vi "Main.vi"   [LabVIEW 2017]
types:
  T1 = cluster{"Note Freq":dbl[], "Note Length":dbl[], "Rest":dbl[]}
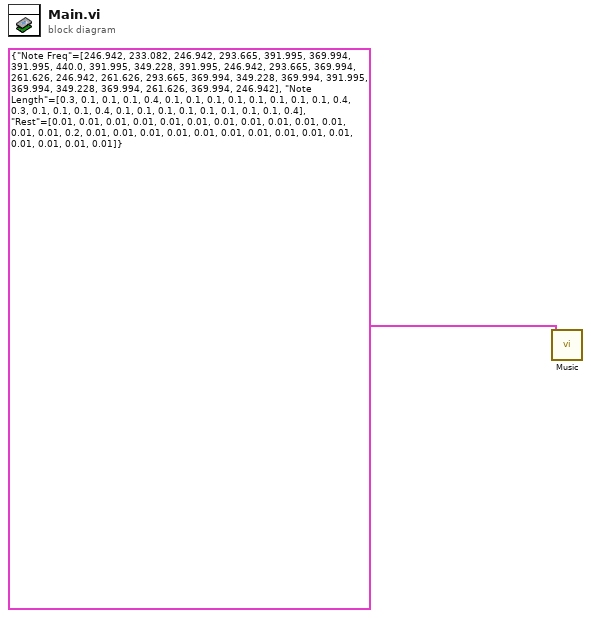
[diagram p0: block diagram]
diagram:
  n1 = call "Music.vi"(11:T1 {"Note Freq"=[246.942, 233.082, 246.942, 293.665, 391.995, 369.994, 391.995, 440.0, 391.995, 349.228, 391.995, 246.942, 293.665, 369.994, 261.626, 246.942, 261.626, 293.665, 369.994, 349.228, 369.994, 391.995, 369.994, 349.228, 369.994, 261.626, 369.994, 246.942], "Note Length"=[0.3, 0.1, 0.1, 0.1, 0.4, 0.1, 0.1, 0.1, 0.1, 0.1, 0.1, 0.1, 0.1, 0.4, 0.3, 0.1, 0.1, 0.1, 0.4, 0.1, 0.1, 0.1, 0.1, 0.1, 0.1, 0.1, 0.1, 0.4], "Rest"=[0.01, 0.01, 0.01, 0.01, 0.01, 0.01, 0.01, 0.01, 0.01, 0.01, 0.01, 0.01, 0.01, 0.2, 0.01, 0.01, 0.01, 0.01, 0.01, 0.01, 0.01, 0.01, 0.01, 0.01, 0.01, 0.01, 0.01, 0.01]}) -> ()  [unwired: 11 in]
